vi "append_line_to_string.vi"(1 "Line to add":string, 2 "String in":string) -> (0 "String out":string)   [LabVIEW 2010]
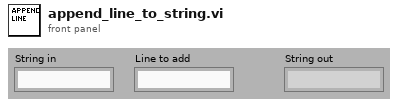
[diagram p1: front panel]
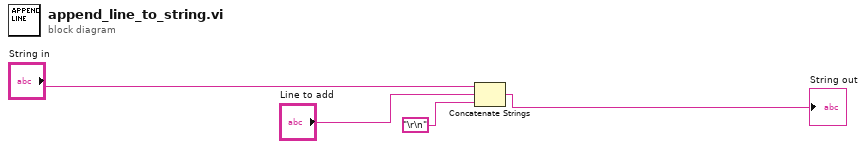
[diagram p0: block diagram]
diagram:
  n1 = Concatenate Strings("String in", "Line to add", "\r\n") -> (→"String out":string)
